vi "PIM Convert 2.0-6.1 to 6.2.vi"(0 "PIM 2.0 - 6.1 Test Parameters":T11={"Stimulus"={"C1 Pwr dBm"=0.0, "C2 Pwr dBm"=0.0, "Power Units"=enum."dBm", "Meas Type"=enum."Frequency", "C1 Freq MHz"=0.0, "C2 Freq MHz"=0.0, "Swept Freq Step"=0}, "Measure"={"IM Order"=0, "Direction"=0, "Averaging"=0, "ALC ON?"=FALSE, "Peak Hold?"=FALSE, "Peak last N"=0, "Ref Level dBm"=0.0, "Ref Units"=enum."dBm", "Num Samples"=0, "Sample units"=enum."Sample(s)", "Update Rate (s)"=0.0, "DUT PORT"=enum."Port 1"}, "Display"={"Power Scale"={"yRange_min"=0, "yRange_max"=0}, "xRange_span"=0}} {"Stimulus"."Swept Freq Step" items=[".2", ".4", "1.0", "2.0"]; "Measure"."Averaging" items=["None", "Minimum", "Normal", "High", "Maximum"]; "Measure"."Direction" items=["Reverse", "Forward", "Auxiliary"]; "Measure"."IM Order" items=["3rd", "5th", "7th", "9th", "11th", "13th", "15th", "17th", "19th", "21st", "23rd", "25th", "27th", "29th", "31st", "33rd"]}) -> (2 "PIM Test Parameters":T1={"Stimulus"={"C1 Pwr dBm"=0.0, "C2 Pwr dBm"=0.0, "Power Units"=enum."dBm", "Meas Type"=enum."Time", "C1 Freq MHz"=0.0, "C2 Freq MHz"=0.0, "Swept Freq Step"=0}, "Measure"={"IM Order"=0, "Direction"=0, "Averaging"=1, "ALC ON?"=TRUE, "Peak Hold?"=TRUE, "Peak last N"=1, "Ref Level dBm"=-100.0, "Ref Units"=enum."dBm", "Num Samples"=1, "Sample units"=enum."Sample(s)", "Update Rate (s)"=0.0, "DUT PORT"=enum."Port 1", "Percent (%)"=100}, "Display"={"Power Scale"={"yRange_min"=-160, "yRange_max"=-60}, "xRange_span"=5}} {"Stimulus"."Swept Freq Step" items=[".2", ".4", "1.0", "2.0"]; "Measure"."Averaging" items=["None", "Minimum", "Normal", "High", "Maximum"]; "Measure"."Direction" items=["Reverse", "Forward", "Auxiliary"]; "Measure"."IM Order" items=["3rd", "5th", "7th", "9th", "11th", "13th", "15th", "17th", "19th", "21st", "23rd", "25th", "27th", "29th", "31st", "33rd"]})   [LabVIEW 2011]
uses:
  TypeDefs/PIM Test Parameters v2.0-6.1.ctl
  TypeDefs/PIM Test Parameters.ctl
  TypeDefs/PIM Stimulus Parameters.ctl
  BPIMCore EXT/HW IO/PIM Sweep Step Size.ctl
  TypeDefs/PIM Measurement Parameters.ctl
  BPIMCore EXT/HW IO/IMOrder.ctl
  BPIMCore EXT/HW IO/MeasMode.ctl
  BPIMCore EXT/HW IO/HW Averaging.ctl
  TypeDefs/PIM Meas Units.ctl
  BPIMCore EXT/HW IO/DUTport.ctl
  TypeDefs/PIM Display Parameters.ctl
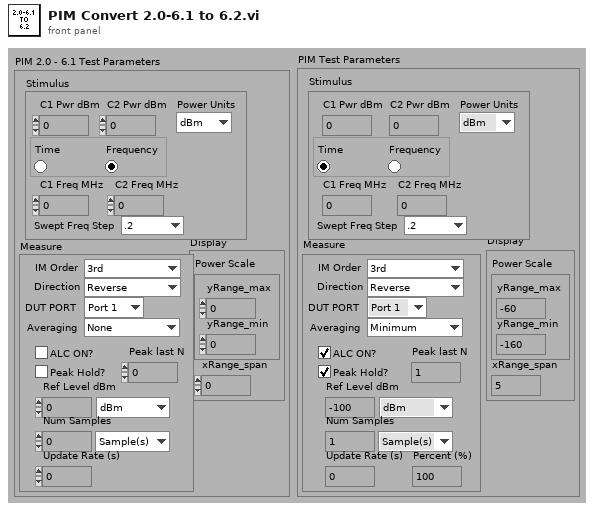
[diagram p1: front panel]
types:
  T1 = typedef "PIM Test Parameters.ctl" = cluster{"Stimulus":T2, "Measure":T4, "Display":T10}
  T2 = typedef "PIM Stimulus Parameters.ctl" = cluster{"C1 Pwr dBm":dbl, "C2 Pwr dBm":dbl, "Power Units":enum16{"dBm", "Watts"}, "Meas Type":enum32{"Time", "Frequency"}, "C1 Freq MHz":dbl, "C2 Freq MHz":dbl, "Swept Freq Step":T3}
  T3 = typedef "PIM Sweep Step Size.ctl" = u16
  T4 = typedef "PIM Measurement Parameters.ctl" = cluster{"IM Order":T5, "Direction":T6, "Averaging":T7, "ALC ON?":bool, "Peak Hold?":bool, "Peak last N":u32, "Ref Level dBm":dbl, "Ref Units":enum16{"dBm", "dBc"}, "Num Samples":u32, "Sample units":T8, "Update Rate (s)":dbl, "DUT PORT":T9, "Percent (%)":u8}
  T5 = typedef "IMOrder.ctl" = u8
  T6 = typedef "MeasMode.ctl" = u16
  T7 = typedef "HW Averaging.ctl" = u16
  T8 = typedef "PIM Meas Units.ctl" = enum16{"Sample(s)", "Second(s)", "Sweep(s)"}
  T9 = typedef "DUTport.ctl" = enum16{"Port 1", "Port 2"}
  T10 = typedef "PIM Display Parameters.ctl" = cluster{"Power Scale":cluster{"yRange_min":i32, "yRange_max":i32}, "xRange_span":u32}
  T11 = typedef "PIM Test Parameters v2.0-6.1.ctl" = cluster{"Stimulus":cluster{"C1 Pwr dBm":dbl, "C2 Pwr dBm":dbl, "Power Units":enum16{"dBm", "Watts"}, "Meas Type":enum32{"Time", "Frequency"}, "C1 Freq MHz":dbl, "C2 Freq MHz":dbl, "Swept Freq Step":u16}, "Measure":cluster{"IM Order":u8, "Direction":u16, "Averaging":u16, "ALC ON?":bool, "Peak Hold?":bool, "Peak last N":u32, "Ref Level dBm":dbl, "Ref Units":enum16{"dBm", "dBc"}, "Num Samples":u32, "Sample units":enum16{"Sample(s)", "Second(s)", "Sweep(s)"}, "Update Rate (s)":dbl, "DUT PORT":enum16{"Port 1", "Port 2"}}, "Display":cluster{"Power Scale":cluster{"yRange_min":i32, "yRange_max":i32}, "xRange_span":u32}}
  T12 = cluster{"C1 Pwr dBm":dbl, "C2 Pwr dBm":dbl, "Power Units":enum16{"dBm", "Watts"}, "Meas Type":enum32{"Time", "Frequency"}, "C1 Freq MHz":dbl, "C2 Freq MHz":dbl, "Swept Freq Step":u16}
  T13 = cluster{"Power Scale":cluster{"yRange_min":i32, "yRange_max":i32}, "xRange_span":u32}
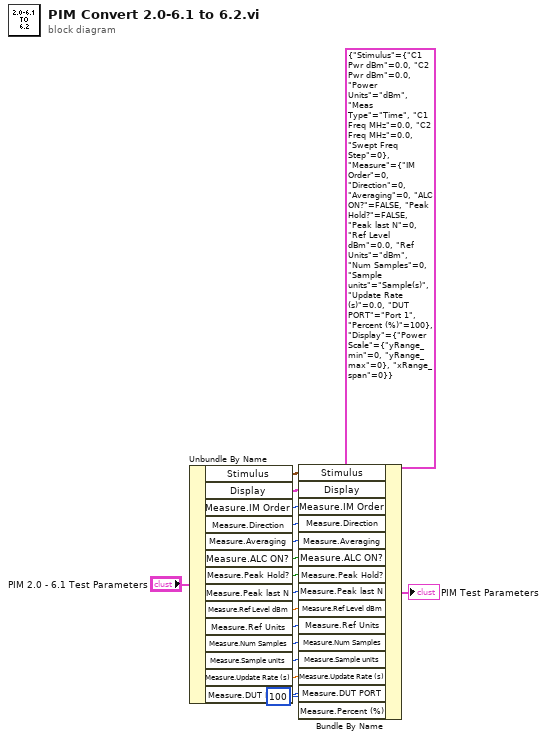
[diagram p0: block diagram]
diagram:
  n1 = Unbundle By Name("PIM 2.0 - 6.1 Test Parameters") -> ("Stimulus"=w14:T12, "Display"=w15:T13, "Measure.IM Order"=w13:u8, "Measure.Direction"=w12:u16, "Measure.Averaging"=w11:u16, "Measure.ALC ON?"=w10:bool, "Measure.Peak Hold?"=w9:bool, "Measure.Peak last N"=w8:u32, "Measure.Ref Level dBm"=w7:dbl, "Measure.Ref Units"=w6:enum16{"dBm", "dBc"}, "Measure.Num Samples"=w5:u32, "Measure.Sample units"=w4:enum16{"Sample(s)", "Second(s)", "Sweep(s)"}, "Measure.Update Rate (s)"=w3:dbl, "Measure.DUT PORT"=w2:enum16{"Port 1", "Port 2"})
  n2 = Bundle By Name(cluster=T1 {"Stimulus"={"C1 Pwr dBm"=0.0, "C2 Pwr dBm"=0.0, "Power Units"=enum."dBm", "Meas Type"=enum."Time", "C1 Freq MHz"=0.0, "C2 Freq MHz"=0.0, "Swept Freq Step"=0}, "Measure"={"IM Order"=0, "Direction"=0, "Averaging"=0, "ALC ON?"=FALSE, "Peak Hold?"=FALSE, "Peak last N"=0, "Ref Level dBm"=0.0, "Ref Units"=enum."dBm", "Num Samples"=0, "Sample units"=enum."Sample(s)", "Update Rate (s)"=0.0, "DUT PORT"=enum."Port 1", "Percent (%)"=100}, "Display"={"Power Scale"={"yRange_min"=0, "yRange_max"=0}, "xRange_span"=0}} ("PIM 1.1 Test Parameters"), "Stimulus"=w14, "Display"=w15, "Measure.IM Order"=w13, "Measure.Direction"=w12, "Measure.Averaging"=w11, "Measure.ALC ON?"=w10, "Measure.Peak Hold?"=w9, "Measure.Peak last N"=w8, "Measure.Ref Level dBm"=w7, "Measure.Ref Units"=w6, "Measure.Num Samples"=w5, "Measure.Sample units"=w4, "Measure.Update Rate (s)"=w3, "Measure.DUT PORT"=w2, "Measure.Percent (%)"=u8 100) -> (→"PIM Test Parameters":T1)
